vi "PS35_GetEmergencyInput.vi"(2 "error in (no error)":errorcluster, 3 "Control unit ID":i32=1 min=1 max=10) -> (0 "error out":errorcluster, 1 "Value-Out":i32)   [LabVIEW 2020]
doc: "PS35_GetEmergencyInput.vi, created: 06.03.2009 alex; last change: 22.10.2019 alex;\n\n<B>FUNCTION:</B> \n\nRead emergency input state.\nAn emergency stop button can be connected at this output. \nIf an emergency stop button is not connected, the short-circuit \njumper has to be used. If the short-circuit jumper is removed \nand if no emergency stop button is attached, the function of \nthe motor power amplifiers is blocked.\n----------------------------------------------------------------------------------------\n<B>INPUT:</B>\n[I32] <B>Control unit ID:</B> control unit index. (Default=1, Range=1...10) \n[CLU] <B>error in</B>\n----------------------------------------------------------------------------------------\n<B>OUTPUT:</B>\n[I32] <B>Value-Out:</B> emergency input state.\n0 – emergency stop button is activated or not connected,\n1 – emergency stop button is not activated, the power amplifiers are switched on.\n[CLU] <B>error out</B>\n----------------------------------------------------------------------------------------\n<B>SUB-VIs:</B>\nPS35_GetReadError.vi\n----------------------------------------------------------------------------------------\n<B>EXT-Calls:</B>\nps35.dll (V2.01)\n----------------------------------------------------------------------------------------"
uses:
  ps35.dll
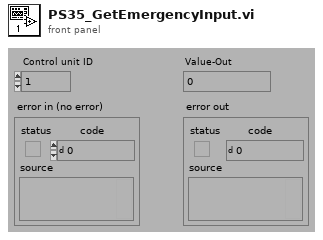
[diagram p1: front panel]
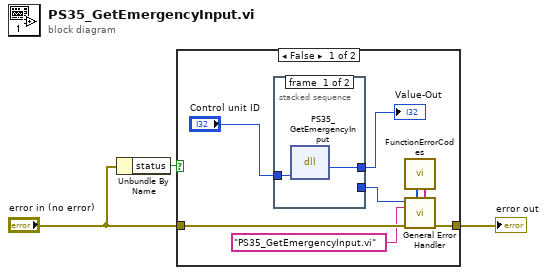
[diagram p0: block diagram]
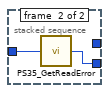
[diagram p2: hidden frame]
diagram:
  n1 = Unbundle By Name("error in (no error)") -> ("status"=w1:bool)
  n2 = case shown="False" w1 {
    tunnel: "error in (no error)" -> [w10 w16]
    tunnel: [w9 w16] -> w3
    frame False {
      n3 = stacked-sequence {
        tunnel: "Control unit ID" -> [w13 w15]
        tunnel: [w12 _] -> w8
        tunnel: [_ w14] -> w7
        frame #0 {
          n4 = dll-call lib="C:/GEECS/Developers Version/source/Device Drivers/OwiSoft/OWISoftOEM/ps35/labview/lv82/ps35.dll" fn="PS35_GetEmergencyInput" label="PS35_Get\nEmergency\nInput"("Index"=w13) -> ("Rückgabetyp"=w12:i32)  [unwired: 4 in, 2 out]
        }
        frame #1 {
          n5 = call "PS35_GetReadError.vi"("Control unit ID"=w15) -> ("Read error"=w14:i32)
        }
      }
      "Value-Out" <- w8
      n6 = call "FunctionErrorCodes.vi"() -> ("[user-defined codes]"=w5:i32[], "[user-defined descriptions]"=w4:string[])  [unwired: 8 in]
      n7 = call <vilib>:"General Error Handler.vi"("[error code] (0)"=w7, "[user-defined codes]"=w5, "[user-defined descriptions]"=w4, "[error source] (\" \")"="PS35_GetEmergencyInput.vi" ("[error source] (\" \")"), "error in (no error)"=w10) -> ("error out"=w9:errorcluster)  [unwired: 6 in, 4 out]
    }
    frame True {
    }
  }
  "error out" <- w3
